vi "Post-Uninstall Custom Action.vi"(10 "Variant":variant) -> (0 "error out":errorcluster)   [LabVIEW 2016]
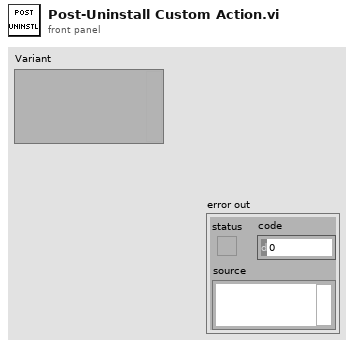
[diagram p1: front panel]
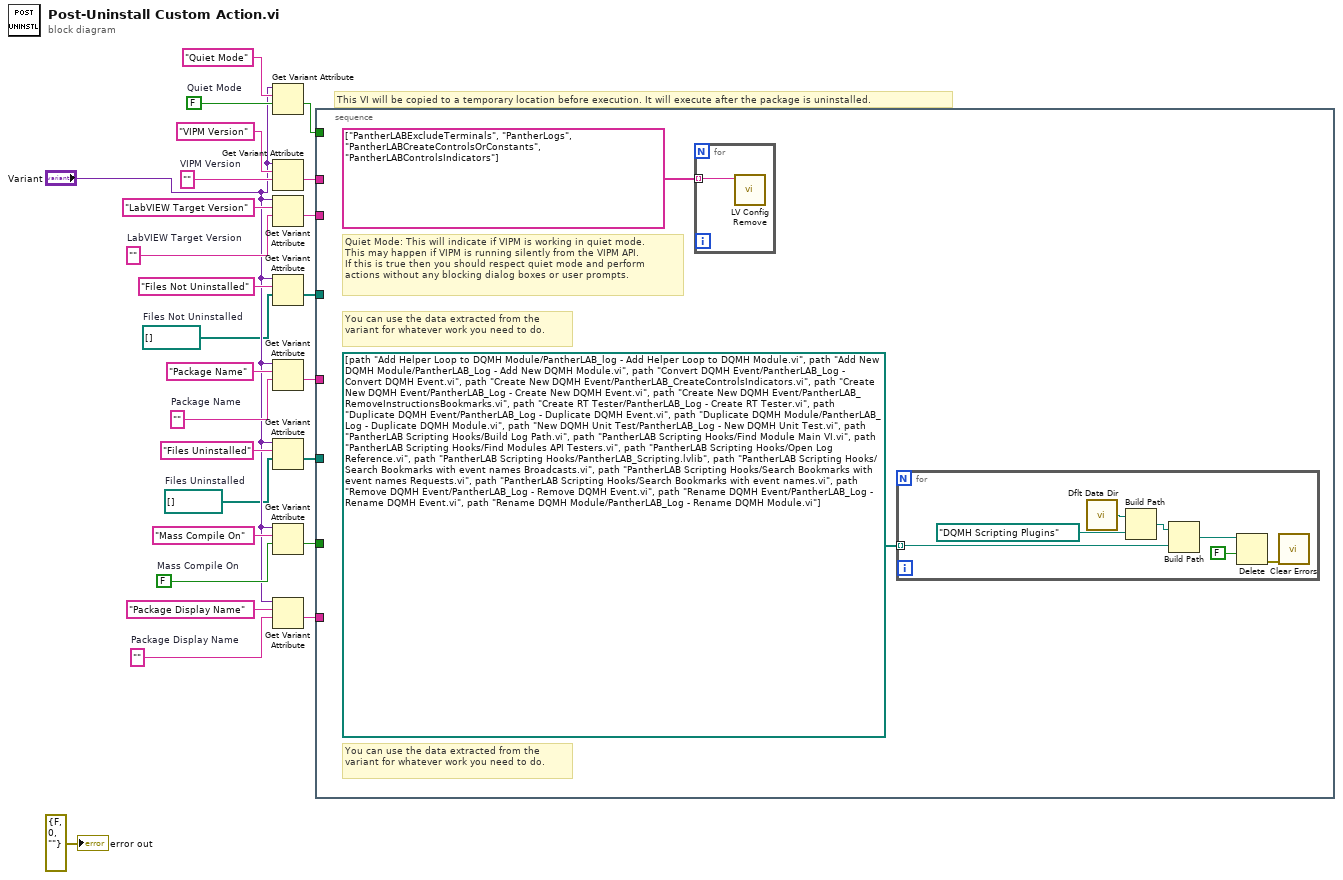
[diagram p0: block diagram]
diagram:
  w1 = path[] []  # Files Not Uninstalled
  w2 = path[] []  # Files Uninstalled
  w8 = FALSE  # Mass Compile On
  w9 = ""  # Package Display Name
  w16 = FALSE  # Quiet Mode
  w19 = ""  # VIPM Version
  w21 = ""  # LabVIEW Target Version
  w23 = ""  # Package Name
  # "This VI will be copied to a temporary location before execution. It will execute after the package is uninstalled."
  n1 = Get Variant Attribute(Variant="Variant", name="Quiet Mode", default value (empty Variant)=w16) -> (value=w11:bool)  [unwired: 1 in, 3 out]
  n2 = Get Variant Attribute(Variant="Variant", name="VIPM Version", default value (empty Variant)=w19) -> (value=w12:string)  [unwired: 1 in, 3 out]
  n3 = Get Variant Attribute(Variant="Variant", name="LabVIEW Target Version", default value (empty Variant)=w21) -> (value=w13:string)  [unwired: 1 in, 3 out]
  n4 = Get Variant Attribute(Variant="Variant", name="Files Not Uninstalled", default value (empty Variant)=w1) -> (value=w6:path[])  [unwired: 1 in, 3 out]
  n5 = Get Variant Attribute(Variant="Variant", name="Package Name", default value (empty Variant)=w23) -> (value=w14:string)  [unwired: 1 in, 3 out]
  n6 = Get Variant Attribute(Variant="Variant", name="Files Uninstalled", default value (empty Variant)=w2) -> (value=w5:path[])  [unwired: 1 in, 3 out]
  n7 = Get Variant Attribute(Variant="Variant", name="Mass Compile On", default value (empty Variant)=w8) -> (value=w10:bool)  [unwired: 1 in, 3 out]
  n8 = Get Variant Attribute(Variant="Variant", name="Package Display Name", default value (empty Variant)=w9) -> (value=w15:string)  [unwired: 1 in, 3 out]
  n9 = stacked-sequence {
    tunnel: w15 -> [_]
    tunnel: w14 -> [_]
    tunnel: w13 -> [_]
    tunnel: w12 -> [_]
    tunnel: w11 -> [_]
    tunnel: w10 -> [_]
    tunnel: w5 -> [_]
    tunnel: w6 -> [_]
    frame #0 {
      # "Quiet Mode: This will indicate if VIPM is working in quiet mode.\nThis may happen if VIPM is running silently from the VIPM API.\nIf this is true then you should respect quiet mode and perform\nactions without any blocking dialog boxes or user prompts."
      # "You can use the data extracted from the variant for whatever work you need to do."
      # "You can use the data extracted from the variant for whatever work you need to do."
      n10 = for {
        tunnel: string[] ["PantherLABExcludeTerminals", "PantherLogs", "PantherLABCreateControlsOrConstants", "PantherLABControlsIndicators"] -> [w29] mode=indexing
        n11 = call <resource>:"LV Config Remove.vi"("key"=w29) -> ()  [unwired: 6 in, 1 out]
      }
      n12 = for {
        tunnel: path[] [path "Add Helper Loop to DQMH Module/PantherLAB_log - Add Helper Loop to DQMH Module.vi", path "Add New DQMH Module/PantherLAB_Log - Add New DQMH Module.vi", path "Convert DQMH Event/PantherLAB_Log - Convert DQMH Event.vi", path "Create New DQMH Event/PantherLAB_CreateControlsIndicators.vi", path "Create New DQMH Event/PantherLAB_Log - Create New DQMH Event.vi", path "Create New DQMH Event/PantherLAB_RemoveInstructionsBookmarks.vi", path "Create RT Tester/PantherLAB_Log - Create RT Tester.vi", path "Duplicate DQMH Event/PantherLAB_Log - Duplicate DQMH Event.vi", path "Duplicate DQMH Module/PantherLAB_Log - Duplicate DQMH Module.vi", path "New DQMH Unit Test/PantherLAB_Log - New DQMH Unit Test.vi", path "PantherLAB Scripting Hooks/Build Log Path.vi", path "PantherLAB Scripting Hooks/Find Module Main VI.vi", path "PantherLAB Scripting Hooks/Find Modules API Testers.vi", path "PantherLAB Scripting Hooks/Open Log Reference.vi", path "PantherLAB Scripting Hooks/PantherLAB_Scripting.lvlib", path "PantherLAB Scripting Hooks/Search Bookmarks with event names Broadcasts.vi", path "PantherLAB Scripting Hooks/Search Bookmarks with event names Requests.vi", path "PantherLAB Scripting Hooks/Search Bookmarks with event names.vi", path "Remove DQMH Event/PantherLAB_Log - Remove DQMH Event.vi", path "Rename DQMH Event/PantherLAB_Log - Rename DQMH Event.vi", path "Rename DQMH Module/PantherLAB_Log - Rename DQMH Module.vi"] ("Files to Delete") -> [w31] mode=indexing
        n13 = call <vilib>:"Dflt Data Dir.vi"() -> ("App:Default Data Directory"=w35:path)
        n14 = Build Path(base path=w35, name or relative path=path "DQMH Scripting Plugins" ("Relative Path from 1 to 2")) -> (appended path=w34:path)
        n15 = Build Path(base path=w34, name or relative path=w31) -> (appended path=w32:path)
        n16 = Delete(path (use dialog)=w32, confirm (F)=FALSE ("overwrite (F)")) -> (error out=w36:errorcluster)  [unwired: 3 in, 2 out]
        n17 = call <vilib>:"Clear Errors.vi"("error in (no error)"=w36) -> ()  [unwired: 5 in, 2 out]
      }
    }
  }
  "error out" <- errorcluster {"status"=FALSE, "code"=0, "source"=""} ("error out")
